vi "FGPaths.vi"(7 "ePathsAction":T1, 8 "error in (no error)":errorcluster, 11 "PathsIn":T2) -> (0 "error out":errorcluster, 3 "PathsOut":T2)   [LabVIEW 2014]
uses:
  typedefs/Paths.ctl
  typedefs/ePathsAction.ctl
  <vilib>/Utility/sysdir.llb/System Directory Type.ctl
  <vilib>/Utility/config.llb/Read Key (Path).vi
  <vilib>/Utility/config.llb/Write Key (Path).vi
  <vilib>/Utility/config.llb/NI_LVConfig.lvlib
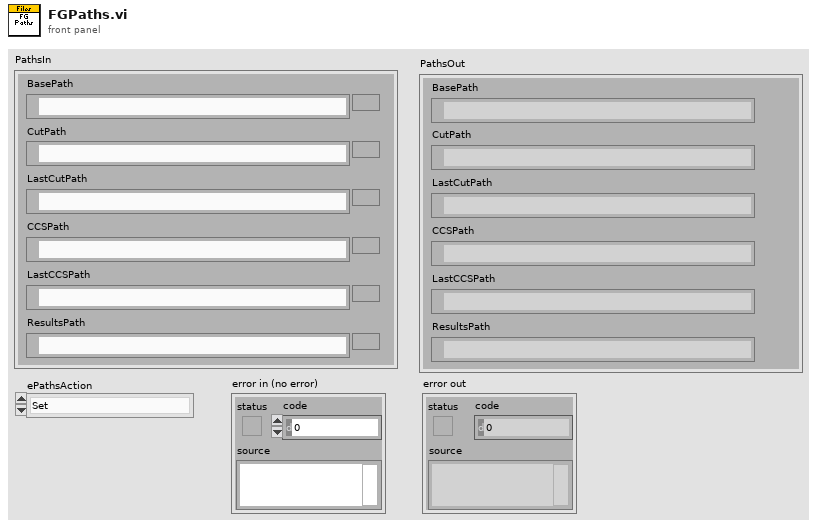
[diagram p1: front panel]
types:
  T1 = typedef "ePathsAction.ctl" = enum16{"Set", "Get", "Load", "Save", "Default", "Exit"}
  T2 = typedef "Paths.ctl" = cluster{"BasePath":path, "CutPath":path, "LastCutPath":path, "CCSPath":path, "LastCCSPath":path, "ResultsPath":path}
  T3 = typedef "NI_LVConfig.lvlib/Config Data RefNum.ctl" = refnum<k1>
  T4 = typedef "System Directory Type.ctl" = i32
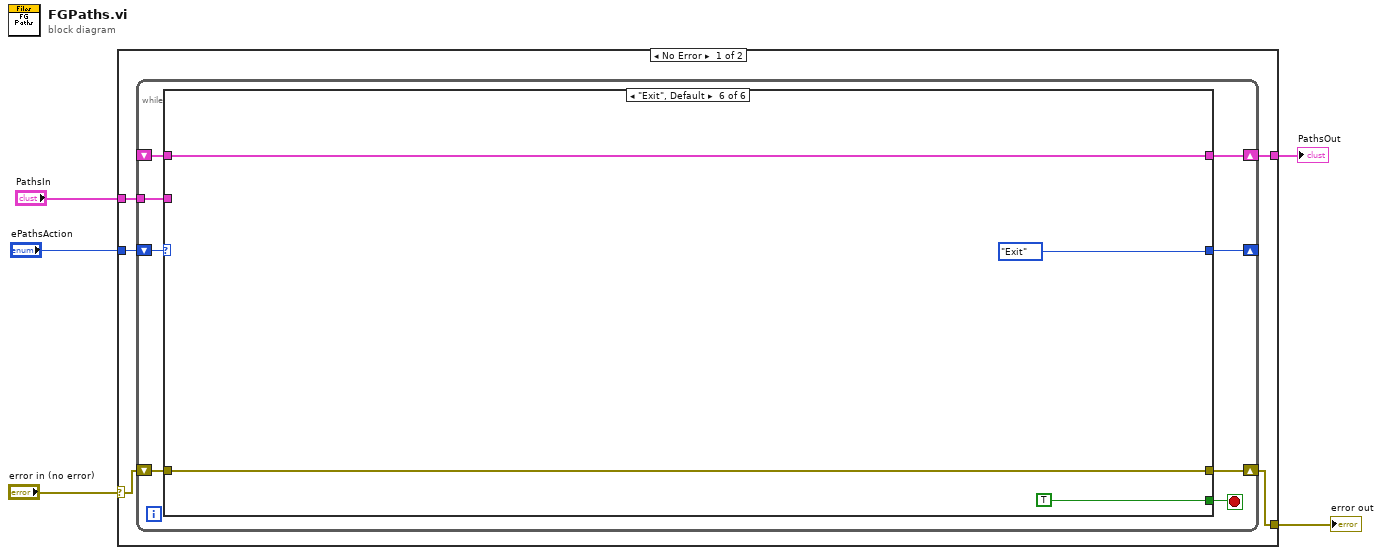
[diagram p0: block diagram]
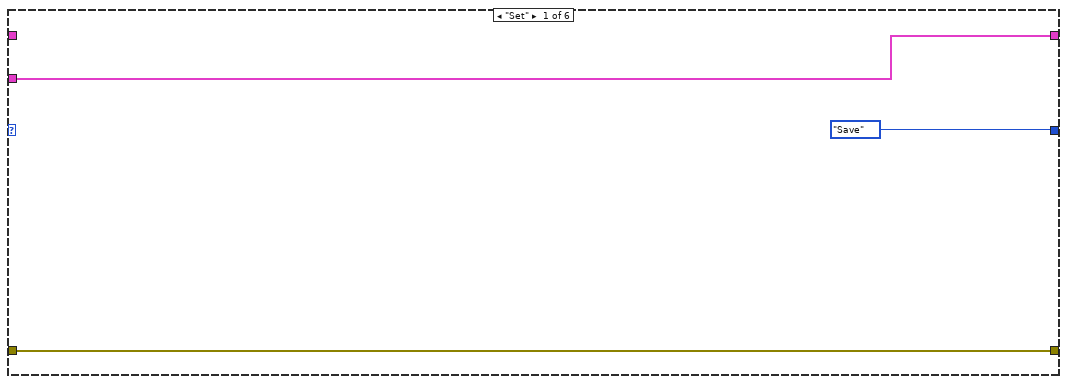
[diagram p2: hidden frame]
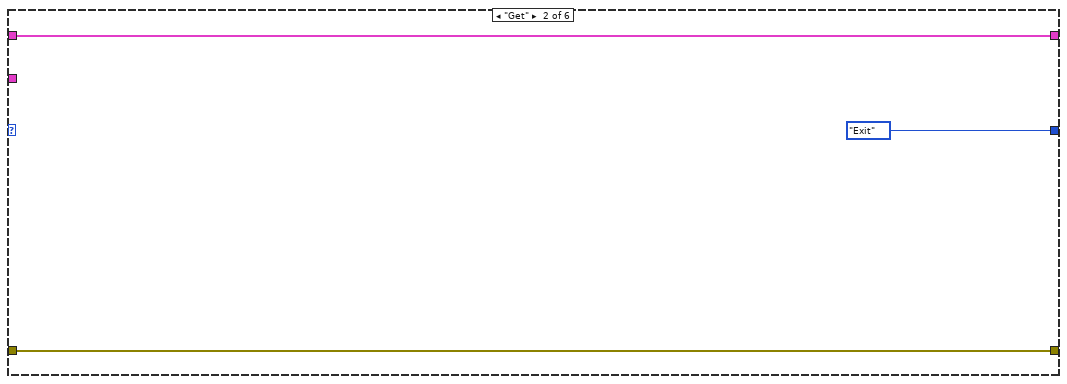
[diagram p3: hidden frame]
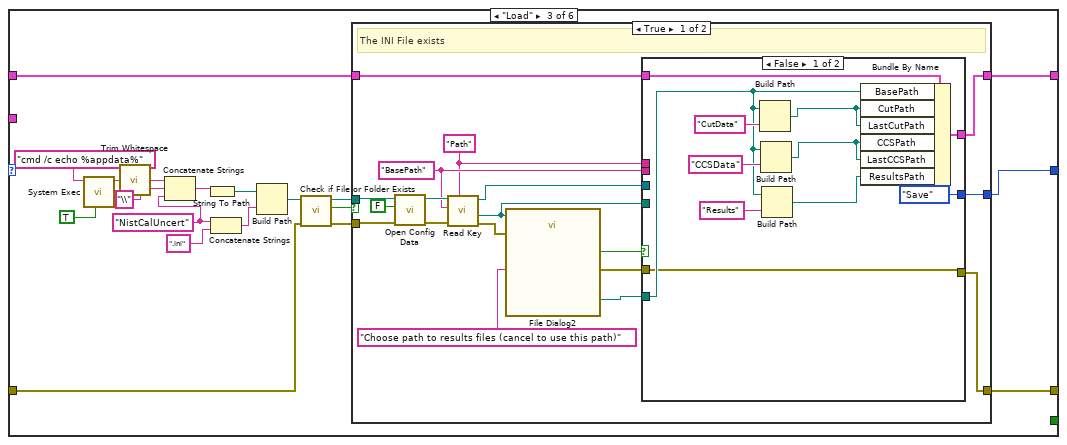
[diagram p4: hidden frame]
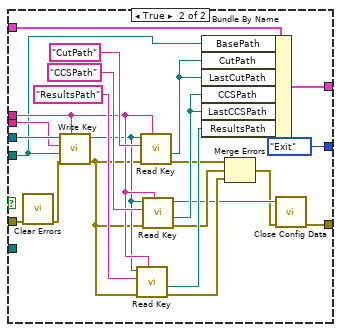
[diagram p5: hidden frame]
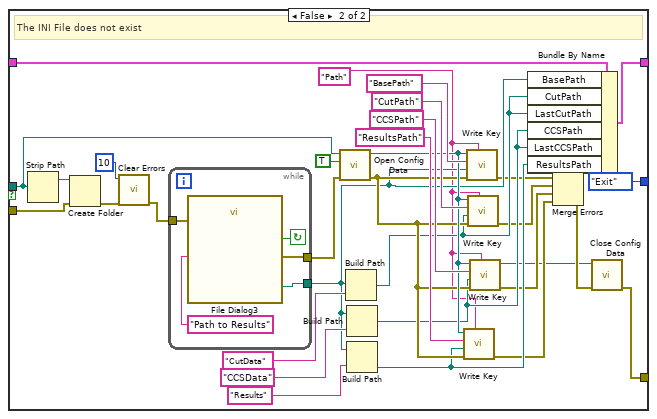
[diagram p6: hidden frame]
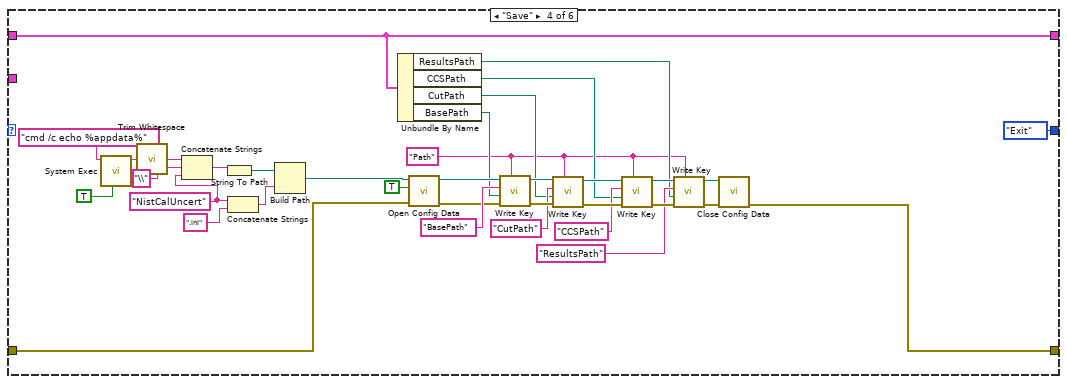
[diagram p7: hidden frame]
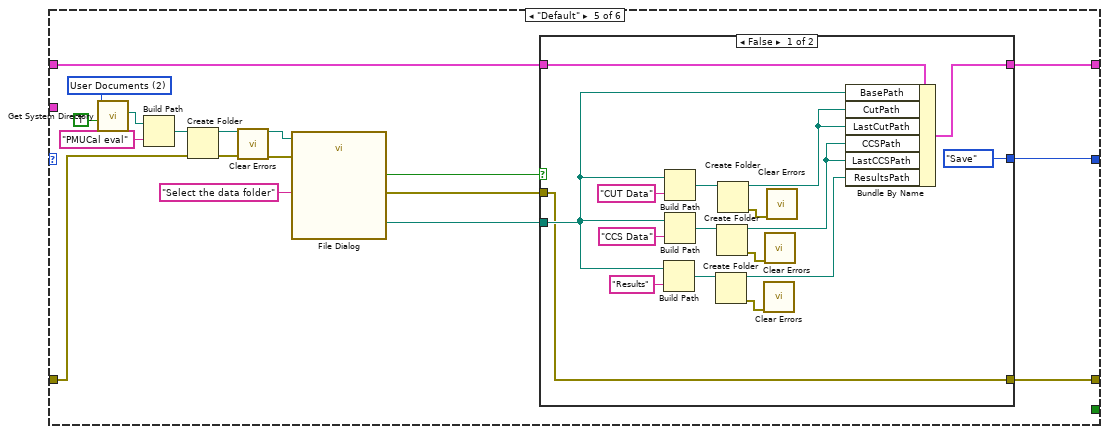
[diagram p8: hidden frame]
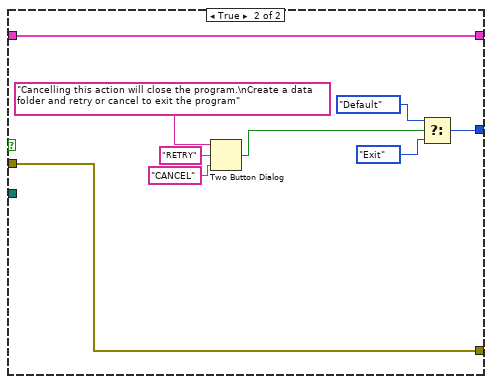
[diagram p9: hidden frame]
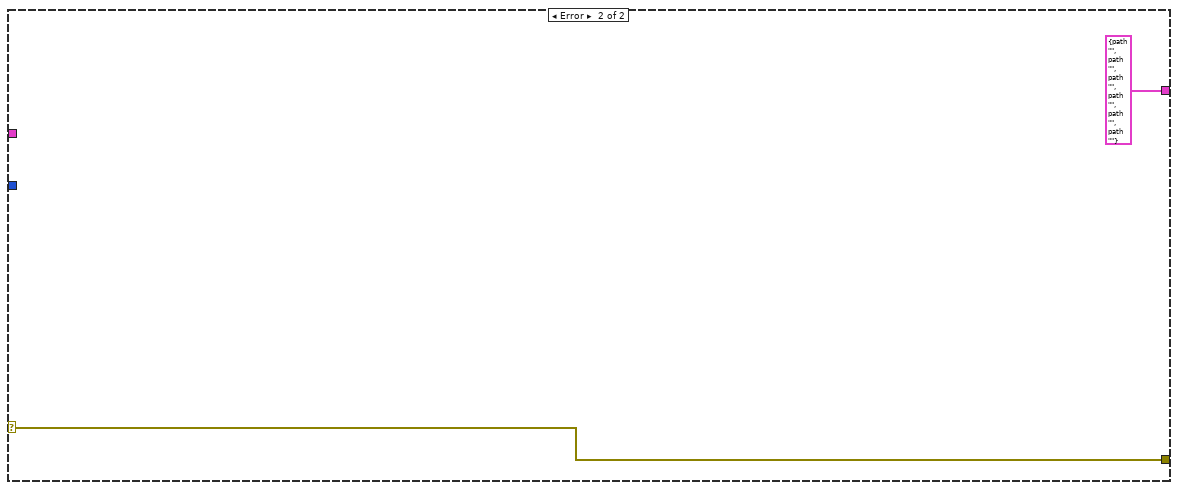
[diagram p10: hidden frame]
diagram:
  n1 = case shown="No Error" "error in (no error)" {
    selector: "error in (no error)" -> [w7 w216]
    tunnel: [w6 w216] -> w4
    tunnel: [w8 T2 {"BasePath"=path "", "CutPath"=path "", "LastCutPath"=path "", "CCSPath"=path "", "LastCCSPath"=path "", "ResultsPath"=path ""} ("PathsOut")] -> w3
    tunnel: "ePathsAction" -> [w10 _]
    tunnel: "PathsIn" -> [w9 _]
    frame No Error {
      n2 = while {
        shift-right: [w16] -> w8
        shift-left: _ -> [w15]
        tunnel: w9 -> [w17]
        shift-right: [w12] -> _
        shift-left: w10 -> [w18]
        shift-right: [w11] -> w6
        shift-left: w7 -> [w14]
        stop <- w13 stop-if-true
        n3 = case shown="\"Exit\", Default" w18 {
          tunnel: w17 -> [w21 _ _ _ _ _]
          tunnel: [w21 w24 w30 w133 w177 w213] -> w16
          tunnel: w15 -> [_ w24 w31 w133 w178 w213]
          tunnel: w14 -> [w19 w22 w29 w135 w175 w211]
          tunnel: [_ _ _ _ _ TRUE] -> w13
          tunnel: [ePathsAction."Save" ("ePathsAction") ePathsAction."Exit" ("ePathsAction") w25 ePathsAction."Exit" ("ePathsAction") w176 ePathsAction."Exit" ("ePathsAction")] -> w12
          tunnel: [w19 w22 w26 w156 w168 w211] -> w11
          frame "Set" {
          }
          frame "Get" {
          }
          frame "Load" {
            w37 = "NistCalUncert" ("string")
            n4 = call <vilib>:"System Exec.vi"("run minimized? (F)"=TRUE, "command line"="cmd /c echo %appdata%") -> ("standard output"=w41:string)  [unwired: 6 in, 3 out]
            n5 = call <vilib>:"Trim Whitespace.vi"("string"=w41) -> ("trimmed string"=w42:string)  [unwired: 1 in]
            n6 = Concatenate Strings(w42, "\\" ("string"), w37) -> (w35:string)
            n7 = String To Path(string=w35) -> (path=w36:path)
            n8 = Concatenate Strings(w37, ".ini" ("string")) -> (w39:string)
            n9 = Build Path(base path=w36, name or relative path=w39) -> (appended path=w32:path)
            n10 = call <vilib>:"Check if File or Folder Exists.vi"("error in (no error)"=w29, "path"=w32) -> ("error out"=w28:errorcluster, "file or folder exists?"=w33:bool, "dup path"=w27:path)  [unwired: 7 in]
            n11 = case shown="True" w33 {
              tunnel: w31 -> [w50 w124]
              tunnel: [w49 w123] -> w30
              tunnel: w28 -> [w59 w121]
              tunnel: w27 -> [w58 w116]
              tunnel: [w48 w99] -> w26
              tunnel: [w44 ePathsAction."Exit" ("ePathsAction")] -> w25
              frame True {
                w53 = "BasePath" ("key")
                w51 = "Path" ("section")
                # "The INI File exists"
                n12 = call <vilib>:"Open Config Data.vi"("error in (no error)"=w59, "create file if necessary (T)"=FALSE, "configuration file path"=w58) -> ("error out"=w57:errorcluster, "refnum"=w61:T3)  [unwired: 6 in, 1 out]
                n13 = call-poly <vilib>:"Read Key.vi"("section"=w51, "error in (no error)"=w57, "key"=w53, "refnum"=w61) -> ("error out"=w56:errorcluster, "value"=w47:path, "refnum out"=w54:T3)  [unwired: 4 in, 1 out]
                n14 = call "File Dialog2"("start path"=w47, "prompt"="Choose path to results files (cancel to use this path)", "error in"=w56) -> ("selected path"=w45:path, "cancelled"=w46:bool, "error out"=w52:errorcluster)  [unwired: 9 in, 1 out]
                n15 = case shown="False" w46 {
                  tunnel: w54 -> [_ w95]
                  tunnel: w53 -> [_ w94]
                  tunnel: w52 -> [w62 w74]
                  tunnel: w51 -> [_ w90]
                  tunnel: w50 -> [w72 w87]
                  tunnel: [w64 w84] -> w49
                  tunnel: [w62 w77] -> w48
                  tunnel: w47 -> [_ w76]
                  tunnel: w45 -> [w68 _]
                  tunnel: [ePathsAction."Save" ("ePathsAction") ePathsAction."Exit" ("ePathsAction")] -> w44
                  frame False {
                    n16 = Build Path(base path=w68, name or relative path="CutData" ("key")) -> (appended path=w67:path)
                    n17 = Build Path(base path=w68, name or relative path="CCSData" ("key")) -> (appended path=w66:path)
                    n18 = Build Path(base path=w68, name or relative path="Results" ("key")) -> (appended path=w65:path)
                    n19 = Bundle By Name(cluster=w72, "BasePath"=w68, "CutPath"=w67, "LastCutPath"=w67, "CCSPath"=w66, "LastCCSPath"=w66, "ResultsPath"=w65) -> (w64:T2)
                  }
                  frame True {
                    n20 = call <vilib>:"Clear Errors.vi"("error in (no error)"=w74) -> ("error out"=w73:errorcluster)  [unwired: 5 in, 1 out]
                    n21 = call-poly <vilib>:"Write Key.vi"("section"=w90, "error in (no error)"=w73, "value"=w76, "key"=w94, "refnum"=w95) -> ("error out"=w88:errorcluster, "refnum out"=w89:T3)  [unwired: 4 in, 1 out]
                    n22 = call-poly <vilib>:"Read Key.vi"("section"=w90, "error in (no error)"=w88, "key"="ResultsPath", "refnum"=w89) -> ("error out"=w80:errorcluster, "value"=w86:path)  [unwired: 4 in, 2 out]
                    n23 = call-poly <vilib>:"Read Key.vi"("section"=w90, "error in (no error)"=w88, "key"="CutPath", "refnum"=w89) -> ("error out"=w82:errorcluster, "value"=w83:path)  [unwired: 4 in, 2 out]
                    n24 = call-poly <vilib>:"Read Key.vi"("section"=w90, "error in (no error)"=w88, "key"="CCSPath", "refnum"=w89) -> ("error out"=w81:errorcluster, "value"=w85:path, "refnum out"=w79:T3)  [unwired: 4 in, 1 out]
                    n25 = Bundle By Name(cluster=w87, "BasePath"=w76, "CutPath"=w83, "LastCutPath"=w83, "CCSPath"=w85, "LastCCSPath"=w85, "ResultsPath"=w86) -> (w84:T2)
                    n26 = Merge Errors(w82, w81, w80) -> (w78:errorcluster)
                    n27 = call <vilib>:"Close Config Data.vi"("error in (no error)"=w78, "refnum"=w79) -> ("error out"=w77:errorcluster)  [unwired: 8 in, 1 out]
                  }
                }
              }
              frame False {
                w100 = "Path" ("section")
                # "The INI File does not exist"
                n28 = Strip Path(path=w116) -> (stripped path=w122:path)  [unwired: 1 out]
                n29 = Create Folder(path (use dialog)=w122, error in=w121) -> (error out=w119:errorcluster)  [unwired: 1 in, 2 out]
                n30 = call <vilib>:"Clear Errors.vi"("error in (no error)"=w119, "specific error code to clear (0: all)"=10) -> ("error out"=w118:errorcluster)  [unwired: 4 in, 1 out]
                n31 = while {
                  tunnel: [w131] -> w108
                  tunnel: w118 -> [w129]
                  tunnel: [w130] -> w115
                  stop <- w128 continue-if-true
                  n32 = call "File Dialog3"("prompt"="Path to Results", "error in"=w129) -> ("selected path"=w131:path, "cancelled"=w128:bool, "error out"=w130:errorcluster)  [unwired: 10 in, 1 out]
                }
                n33 = call <vilib>:"Open Config Data.vi"("error in (no error)"=w115, "create file if necessary (T)"=TRUE, "configuration file path"=w116) -> ("error out"=w112:errorcluster, "refnum"=w113:T3)  [unwired: 6 in, 1 out]
                n34 = Build Path(base path=w108, name or relative path="CutData" ("key")) -> (appended path=w106:path)
                n35 = Build Path(base path=w108, name or relative path="CCSData" ("key")) -> (appended path=w107:path)
                n36 = Build Path(base path=w108, name or relative path="Results" ("key")) -> (appended path=w105:path)
                n37 = call-poly <vilib>:"Write Key.vi"("section"=w100, "error in (no error)"=w112, "value"=w105, "key"="ResultsPath", "refnum"=w113) -> ("error out"=w101:errorcluster)  [unwired: 4 in, 2 out]
                n38 = call-poly <vilib>:"Write Key.vi"("section"=w100, "error in (no error)"=w112, "value"=w108, "key"="BasePath", "refnum"=w113) -> ("error out"=w104:errorcluster)  [unwired: 4 in, 2 out]
                n39 = call-poly <vilib>:"Write Key.vi"("section"=w100, "error in (no error)"=w112, "value"=w106, "key"="CutPath", "refnum"=w113) -> ("error out"=w103:errorcluster)  [unwired: 4 in, 2 out]
                n40 = call-poly <vilib>:"Write Key.vi"("section"=w100, "error in (no error)"=w112, "value"=w107, "key"="CCSPath", "refnum"=w113) -> ("error out"=w102:errorcluster, "refnum out"=w97:T3)  [unwired: 4 in, 1 out]
                n41 = Bundle By Name(cluster=w124, "BasePath"=w108, "CutPath"=w106, "LastCutPath"=w106, "CCSPath"=w107, "LastCCSPath"=w107, "ResultsPath"=w105) -> (w123:T2)
                n42 = Merge Errors(w104, w103, w102, w101) -> (w98:errorcluster)
                n43 = call <vilib>:"Close Config Data.vi"("error in (no error)"=w98, "refnum"=w97) -> ("error out"=w99:errorcluster)  [unwired: 8 in, 1 out]
              }
            }
          }
          frame "Save" {
            w136 = "Path" ("section")
            w160 = "NistCalUncert" ("string")
            n44 = call <vilib>:"System Exec.vi"("run minimized? (F)"=TRUE, "command line"="cmd /c echo %appdata%") -> ("standard output"=w164:string)  [unwired: 6 in, 3 out]
            n45 = call <vilib>:"Trim Whitespace.vi"("string"=w164) -> ("trimmed string"=w165:string)  [unwired: 1 in]
            n46 = Concatenate Strings(w165, "\\" ("string"), w160) -> (w158:string)
            n47 = String To Path(string=w158) -> (path=w159:path)
            n48 = Concatenate Strings(w160, ".ini" ("string")) -> (w162:string)
            n49 = Build Path(base path=w159, name or relative path=w162) -> (appended path=w134:path)
            n50 = Unbundle By Name(w133) -> ("ResultsPath"=w139:path, "CCSPath"=w143:path, "CutPath"=w147:path, "BasePath"=w152:path)
            n51 = call <vilib>:"Open Config Data.vi"("error in (no error)"=w135, "create file if necessary (T)"=TRUE, "configuration file path"=w134) -> ("error out"=w151:errorcluster, "refnum"=w153:T3)  [unwired: 6 in, 1 out]
            n52 = call-poly <vilib>:"Write Key.vi"("section"=w136, "error in (no error)"=w151, "value"=w152, "key"="BasePath", "refnum"=w153) -> ("error out"=w149:errorcluster, "refnum out"=w150:T3)  [unwired: 4 in, 1 out]
            n53 = call-poly <vilib>:"Write Key.vi"("section"=w136, "error in (no error)"=w149, "value"=w147, "key"="CutPath", "refnum"=w150) -> ("error out"=w145:errorcluster, "refnum out"=w146:T3)  [unwired: 4 in, 1 out]
            n54 = call-poly <vilib>:"Write Key.vi"("section"=w136, "error in (no error)"=w145, "value"=w143, "key"="CCSPath", "refnum"=w146) -> ("error out"=w141:errorcluster, "refnum out"=w142:T3)  [unwired: 4 in, 1 out]
            n55 = call-poly <vilib>:"Write Key.vi"("section"=w136, "error in (no error)"=w141, "value"=w139, "key"="ResultsPath", "refnum"=w142) -> ("error out"=w137:errorcluster, "refnum out"=w138:T3)  [unwired: 4 in, 1 out]
            n56 = call <vilib>:"Close Config Data.vi"("error in (no error)"=w137, "refnum"=w138) -> ("error out"=w156:errorcluster)  [unwired: 8 in, 1 out]
          }
          frame "Default" {
            w184 = T4 2 items=["User Home"=0, "User Desktop"=1, "User Documents"=2, "User Application Data"=3, "User Preferences"=4, "User Temporary"=5, "Public Documents"=6, "Public Application Data"=7, "Public Preferences"=8, "Public Cache"=13, "System Core Libraries"=9, "System Installed Libraries"=10, "Application Files"=11, "Boot Volume Root"=12] ("system directory type")
            n57 = call <vilib>:"Get System Directory.vi"("create directory if not found? (F)"=TRUE, "system directory type"=w184) -> ("system directory"=w182:path)  [unwired: 9 in]
            n58 = Build Path(base path=w182, name or relative path="PMUCal eval") -> (appended path=w180:path)
            n59 = Create Folder(path (use dialog)=w180, error in=w175) -> (created path=w173:path, error out=w179:errorcluster)  [unwired: 1 in, 1 out]
            n60 = call <vilib>:"Clear Errors.vi"("error in (no error)"=w179) -> ("error out"=w174:errorcluster)  [unwired: 5 in, 1 out]
            n61 = call "File Dialog"("start path"=w173, "prompt"="Select the data folder", "error in"=w174) -> ("selected path"=w172:path, "cancelled"=w170:bool, "error out"=w169:errorcluster)  [unwired: 9 in, 1 out]
            n62 = case shown="False" w170 {
              tunnel: w178 -> [w201 w202]
              tunnel: [w198 w202] -> w177
              tunnel: [ePathsAction."Save" ("ePathsAction") w206] -> w176
              tunnel: w172 -> [w186 _]
              tunnel: w169 -> [w185 w203]
              tunnel: [w185 w203] -> w168
              frame False {
                n63 = Build Path(base path=w186, name or relative path="Results") -> (appended path=w190:path)
                n64 = Build Path(base path=w186, name or relative path="CUT Data") -> (appended path=w195:path)
                n65 = Build Path(base path=w186, name or relative path="CCS Data") -> (appended path=w197:path)
                n66 = Create Folder(path (use dialog)=w190) -> (created path=w188:path, error out=w191:errorcluster)  [unwired: 2 in, 1 out]
                n67 = Create Folder(path (use dialog)=w197) -> (created path=w196:path, error out=w193:errorcluster)  [unwired: 2 in, 1 out]
                n68 = Create Folder(path (use dialog)=w195) -> (created path=w194:path, error out=w192:errorcluster)  [unwired: 2 in, 1 out]
                n69 = call <vilib>:"Clear Errors.vi"("error in (no error)"=w191) -> ()  [unwired: 5 in, 2 out]
                n70 = call <vilib>:"Clear Errors.vi"("error in (no error)"=w193) -> ()  [unwired: 5 in, 2 out]
                n71 = call <vilib>:"Clear Errors.vi"("error in (no error)"=w192) -> ()  [unwired: 5 in, 2 out]
                n72 = Bundle By Name(cluster=w201, "BasePath"=w186, "CutPath"=w194, "LastCutPath"=w194, "CCSPath"=w196, "LastCCSPath"=w196, "ResultsPath"=w188) -> (w198:T2)
              }
              frame True {
                n73 = Two Button Dialog(message="Cancelling this action will close the program.\nCreate a data folder and retry or cancel to exit the program", 1:"CANCEL" ("F button name (\"Cancel\")"), 2:"RETRY" ("T button name (\"OK\")")) -> (T button?=w204:bool)
                n74 = Select(t=ePathsAction."Default" ("ePathsAction"), s=w204, f=ePathsAction."Exit" ("ePathsAction")) -> (s? t:f=w206:T1)
              }
            }
          }
          frame "Exit", Default {
          }
        }
      }
    }
    frame Error {
    }
  }
  "PathsOut" <- w3
  "error out" <- w4
